vi "Rendevouz.vi"() -> ()   [LabVIEW 2016]
panel:
  out "number (0 to 1) 2":dbl(graph)
  out "Numeric Control 2":i32
  out "Numeric Control":i32
  in  "Stop Button":bool
  out "number (0 to 1)":dbl(graph)
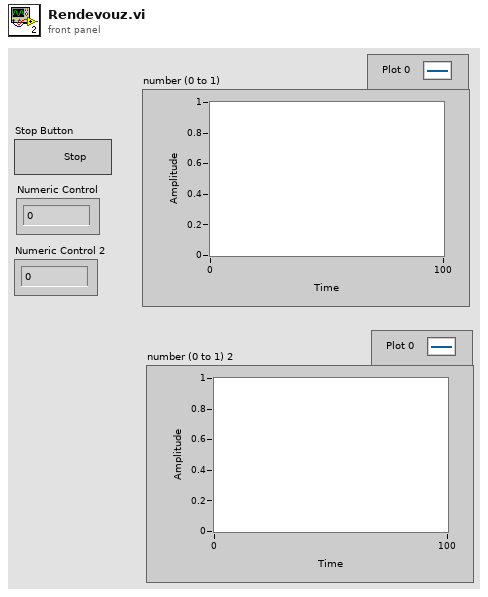
[diagram p1: front panel]
types:
  T1 = typedef "Rendezvous RefNum" = refnum<k1>
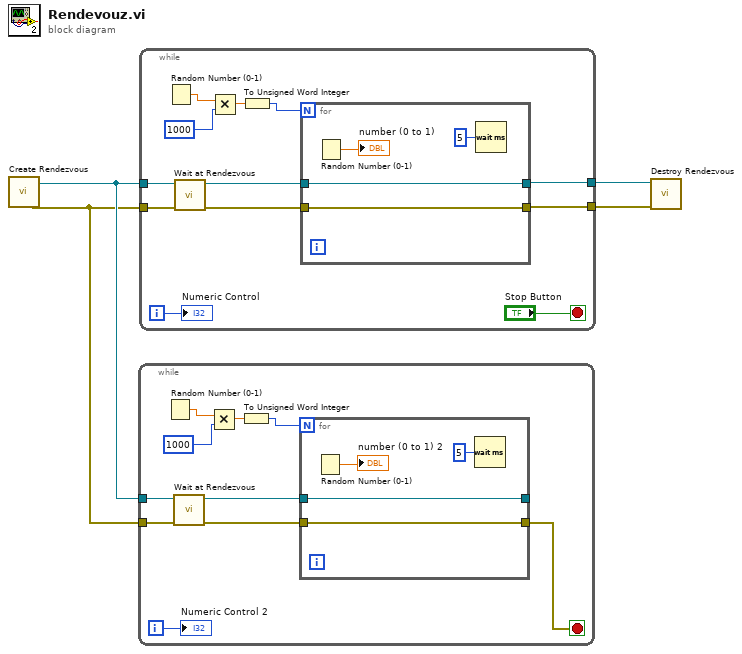
[diagram p0: block diagram]
diagram:
  n1 = call <vilib>:"Create Rendezvous.vi"() -> ("error out"=w3:errorcluster, "rendezvous"=w4:T1)  [unwired: 5 in, 1 out]
  n2 = while {
    tunnel: w4 -> [w7]
    tunnel: w3 -> [w6]
    i -> [w10]
    stop <- w5 stop-if-true
    n3 = Random Number (0-1)() -> (number: 0 to 1=w11:dbl)
    n4 = call <vilib>:"Wait at Rendezvous.vi"("error in (no error)"=w6, "rendezvous"=w7) -> ("error out"=w8:errorcluster, "rendezvous out"=w9:T1)  [unwired: 3 in, 1 out]
    n5 = Multiply(x=w11, y=1000) -> (x*y=w14:dbl)
    n6 = To Unsigned Word Integer(number=w14) -> (unsigned 16bit integer=w13:u16)
    n7 = for {
      N: w13 -> [_]
      tunnel: w9 -> [w16]
      tunnel: w8 -> [w15]
      tunnel: [w16] -> _
      tunnel: [w15] -> w5
      n8 = Random Number (0-1)() -> (number: 0 to 1=→"number (0 to 1) 2":dbl)
      n9 = Wait (ms)(milliseconds to wait=u32 5) -> ()  [unwired: 1 out]
    }
    "Numeric Control 2" <- w10
  }
  n10 = while {
    tunnel: w4 -> [w22]
    tunnel: w3 -> [w21]
    tunnel: [w20] -> w2
    tunnel: [w19] -> w1
    i -> [w25]
    stop <- "Stop Button" stop-if-true
    n11 = Random Number (0-1)() -> (number: 0 to 1=w27:dbl)
    n12 = call <vilib>:"Wait at Rendezvous.vi"("error in (no error)"=w21, "rendezvous"=w22) -> ("error out"=w23:errorcluster, "rendezvous out"=w24:T1)  [unwired: 3 in, 1 out]
    n13 = Multiply(x=w27, y=1000) -> (x*y=w30:dbl)
    n14 = To Unsigned Word Integer(number=w30) -> (unsigned 16bit integer=w29:u16)
    n15 = for {
      N: w29 -> [_]
      tunnel: w24 -> [w32]
      tunnel: w23 -> [w31]
      tunnel: [w32] -> w20
      tunnel: [w31] -> w19
      n16 = Random Number (0-1)() -> (number: 0 to 1=→"number (0 to 1)":dbl)
      n17 = Wait (ms)(milliseconds to wait=u32 5) -> ()  [unwired: 1 out]
    }
    "Numeric Control" <- w25
  }
  n18 = call <vilib>:"Destroy Rendezvous.vi"("error in (no error)"=w1, "rendezvous"=w2) -> ()  [unwired: 4 in, 2 out]
